vi "relay_project.vi"() -> ()   [LabVIEW 2020]
uses:
  <vilib>/LabVIEW Interface for Arduino/Type Defs/Board Type.ctl
  <vilib>/LabVIEW Interface for Arduino/LabVIEW Interface for Arduino.lvlib
panel:
  in  "stop":bool
  out "Value":u8
  in  "Vertical Slide Switch":bool
  in  "Digital I/O Pin (0)":u8
  in  "VISA resource":refnum<visa-resource-name>
  # "On/OFF Relay Switch Project"
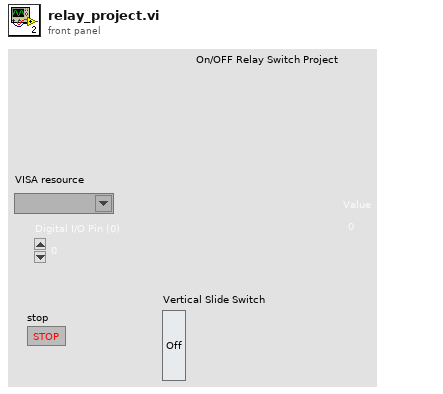
[diagram p1: front panel]
types:
  T1 = typedef "LabVIEW Interface for Arduino.lvlib/Board Type.ctl" = enum16{"Uno", "Dimuelanove w/Atmega 328", "Mega 2560"}
  T2 = typedef "LabVIEW Interface for Arduino.lvlib/Arduino Resource.ctl" = cluster{"VISA resource":refnum<visa-resource-name>, "Board Type":T1, "Connection Type":enum8{"USB / Serial"}, "Bytes Per Packet (15)":u8}
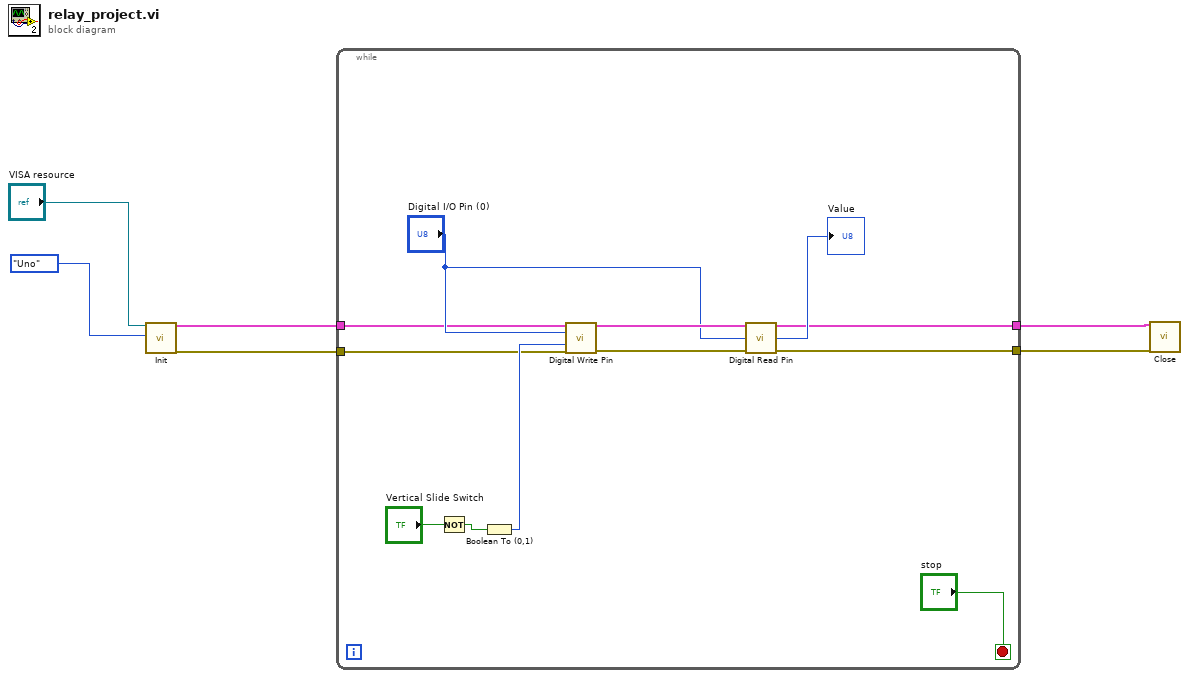
[diagram p0: block diagram]
diagram:
  n1 = call <vilib>:"Init.vi"("VISA resource"="VISA resource", "Board Type (Uno)"=Board_Type."Uno") -> ("Arduino Resource"=w4:T2, "error out"=w3:errorcluster)  [unwired: 16 in]
  n2 = while {
    tunnel: w4 -> [w11]
    tunnel: w3 -> [w9]
    tunnel: [w8] -> w2
    tunnel: [w7] -> w1
    stop <- "stop" stop-if-true
    n3 = Not(x="Vertical Slide Switch") -> (.not. x?=w13:bool)
    n4 = Boolean To (0,1)(Boolean=w13) -> (0, 1=w10:i16)
    n5 = call <vilib>:"Digital Write Pin.vi"("Arduino Resource"=w11, "Digital I/O Pin (0)"="Digital I/O Pin (0)", "Value (0)"=w10, "error in"=w9) -> ("Arduino Resource"=w18:T2, "error out"=w17:errorcluster)  [unwired: 10 in]
    n6 = call <vilib>:"Digital Read Pin.vi"("Arduino Resource"=w18, "Digital I/O Pin (0)"="Digital I/O Pin (0)", "error in"=w17) -> ("Arduino Resource"=w8:T2, "Value"=→"Value":u8, "error out"=w7:errorcluster)  [unwired: 10 in]
  }
  n7 = call <vilib>:"Close.vi"("Arduino Resource"=w2, "error in"=w1) -> ()  [unwired: 13 in, 1 out]
